vi "Fixup Time.vi"(10 "dt (s) in":dbl, 11 "Initialize?:":bool) -> (2 "dt (s) out":dbl)   [LabVIEW 2020]
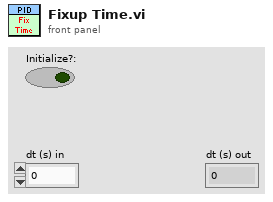
[diagram p1: front panel]
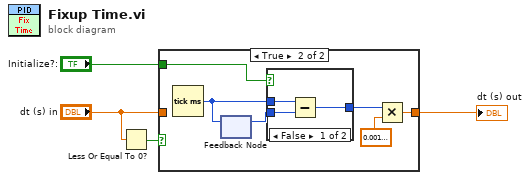
[diagram p0: block diagram]
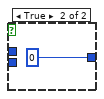
[diagram p3: hidden frame]
diagram:
  n1 = Less Or Equal To 0?(x="dt (s) in") -> (x <= 0?=w2:bool)
  n2 = case shown="True" w2 {
    tunnel: [w5 w10] -> w4
    tunnel: "dt (s) in" -> [w5 _]
    tunnel: "Initialize?:" -> [_ w9]
    frame False {
    }
    frame True {
      n3 = Tick Count (ms)() -> (millisecond timer value=w6:u32)
      n4 = feedback #1() -> (w7:u32)  [unwired: 1 in]
      n5 = feedback-in #1(w6) -> ()
      n6 = case shown="False" w9 {
        tunnel: [w14 u32 0] -> w8
        tunnel: w7 -> [w13 _]
        tunnel: w6 -> [w12 _]
        frame False {
          n7 = Subtract(x=w12, y=w13) -> (x-y=w14:u32)
        }
        frame True {
        }
      }
      n8 = Multiply(x=w8, y=0.0010000000474974513) -> (x*y=w10:dbl)
    }
  }
  "dt (s) out" <- w4
